vi "Station Read Station Initialize Item.vi"(8 "error in (no error)":errorcluster, 9 "Column ID.":T1, 10 "Row ID.":T2(ring), 11 "Station in":refnum<class "Station.lvclass">) -> (0 "error out":errorcluster, 1 "Station Initialize Row Data":string[](array[string]), 2 "Requested Item":string, 3 "Station out":refnum<class "Station.lvclass">)   [LabVIEW 2018, in "Station.lvclass"]
uses:
  Station.lvclass
  Controls/Column ID Select.ctl
  Station.lvclass/Station.ctl
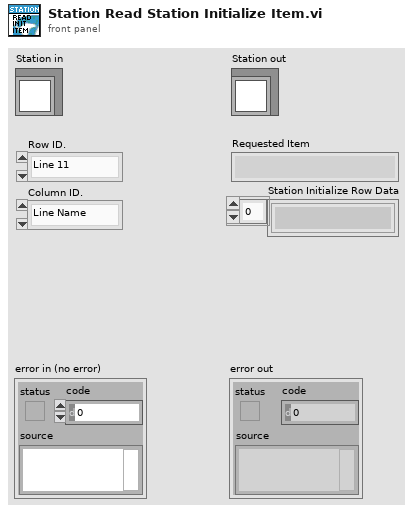
[diagram p1: front panel]
types:
  T1 = typedef "Column ID Select.ctl" = enum16{"Line Name", "Rack ID", "Instrument Mnemonic", "Component Mnemonic", "Subsystme Mnemonic", "Instrument Availability", "IP Address", "Sub Address", "Model Number", "Firmware Revision", "Expected Options", "Required Options", "Excluded Options"}
  T2 = enum16{"Line 11", "Line 12", "Line 13", "Line 14", "Line 15", "Line 16", "Line 17", "Line 18", "Line 19", "Line 19a", "Line 19b", "Line 19c", "Line 19d", "Line 19e", "Line 20", "Line 20a", "Line 20b", "Line 20c", "Line 20d", "Line 21", "Line 22", "Line 22a", "Line 22b", "Line 22c", "Line 22d", "Line 23", "Line 23a", "Line 23b", "Line 23c", "Line 24", "Line 25", "Line 26", "Line 27", "Line 28", "Line 29", "Line 30"}
  T3 = typedef "Station Initialize Data.ctl" = string[][]
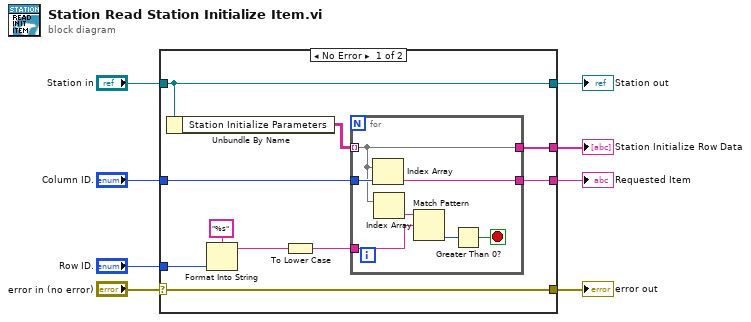
[diagram p0: block diagram]
diagram:
  n1 = case shown="No Error" "error in (no error)" {
    selector: "error in (no error)" -> [w18 w27]
    tunnel: [w18 w27] -> w3
    tunnel: "Row ID." -> [w16 _]
    tunnel: "Column ID." -> [w14 _]
    tunnel: [w13 _] -> w6
    tunnel: [w12 _] -> w5
    tunnel: [w10 w26] -> w2
    tunnel: "Station in" -> [w10 w26]
    frame No Error {
      n2 = Unbundle By Name(w10) -> ("Station Initialize Parameters"=w9:T3)
      n3 = Format Into String(format string="%s", w16) -> (resulting string=w15:string)  [unwired: 2 in, 1 out]
      n4 = To Lower Case(string=w15) -> (all lower case string=w11:string)
      n5 = for {
        tunnel: w9 -> [w19] mode=indexing
        tunnel: w11 -> [w24]
        tunnel: w14 -> [w21]
        tunnel: [w20] -> w13
        tunnel: [w19] -> w12
        stop <- w22 stop-if-true
        n6 = Index Array(array=w19, index=w21) -> (element=w20:string)
        n7 = Index Array(array=w19) -> (element=w25:string)  [unwired: 1 in]
        n8 = Match Pattern(string=w25, regular expression=w24) -> (offset past match=w23:i32)  [unwired: 1 in, 3 out]
        n9 = Greater Than 0?(x=w23) -> (x > 0?=w22:bool)
      }
    }
    frame Error {
    }
  }
  "error out" <- w3
  "Station out" <- w2
  "Requested Item" <- w6
  "Station Initialize Row Data" <- w5
